vi "add_SetSonarLights_roslv.vi"(4 "Lights":T1, 5 "msg in":string) -> (2 "msg out":string)   [LabVIEW 2014]
doc: "Translates LabVIEW indicator for setting sonar lights into a message that can be interpretted in ROS"
uses:
  std_msgs/subs/u16Scalar_roslv.vi
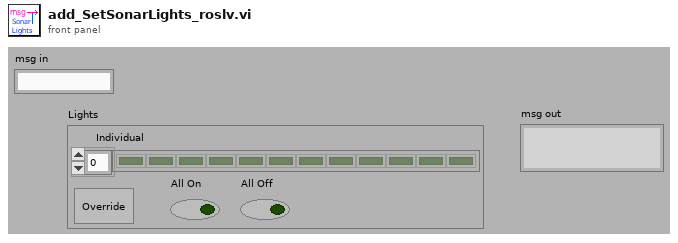
[diagram p1: front panel]
types:
  T1 = cluster{"Behavior":bool, "All On":bool, "All Off":bool, "Individual":bool[]}
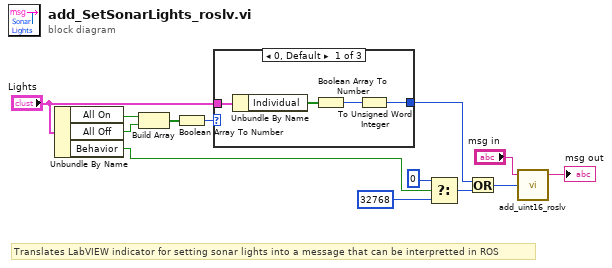
[diagram p0: block diagram]
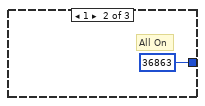
[diagram p2: hidden frame]
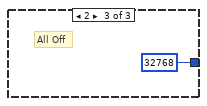
[diagram p3: hidden frame]
diagram:
  # "Translates LabVIEW indicator for setting sonar lights into a message that can be interpretted in ROS"
  n1 = Unbundle By Name("Lights") -> ("All On"=w9:bool, "All Off"=w8:bool, "Behavior"=w6:bool)
  n2 = Build Array(w9, w8) -> (w1:bool[])
  n3 = Boolean Array To Number(Boolean array=w1) -> (number=w7:u32)
  n4 = case shown="0, Default" w7 {
    tunnel: "Lights" -> [w17 _ _]
    tunnel: [w14 u16 36863 u16 32768 ("f")] -> w2
    frame 0, Default {
      n5 = Unbundle By Name(w17) -> ("Individual"=w16:bool[])
      n6 = Boolean Array To Number(Boolean array=w16) -> (number=w15:u32)
      n7 = To Unsigned Word Integer(number=w15) -> (unsigned 16bit integer=w14:u16)
    }
    frame 1 {
      # "All On"
    }
    frame 2 {
      # "All Off"
    }
  }
  n8 = Select(t=u16 0, s=w6, f=u16 32768) -> (s? t:f=w3:u16)
  n9 = Or(x=w2, y=w3) -> (x .or. y?=w12:u16)
  n10 = call-poly "add_uint16_roslv.vi"("Numeric"=w12, "msg in"="msg in") -> ("msg out"=→"msg out":string)  [unwired: 3 in]
